vi "PathOff.vi"(11 "Path":T2) -> (3 "PathOut":T2)   [LabVIEW 2014]
uses:
  TypeDefs/Point2DwSlope.ctl
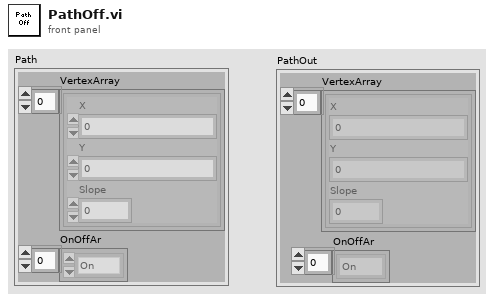
[diagram p1: front panel]
types:
  T1 = typedef "Point2DwSlope.ctl" = cluster{"X":sgl, "Y":sgl, "Slope":dbl}
  T2 = cluster{"VertexArray":T1[], "OnOffAr":enum16{"On", "Off"}[]}
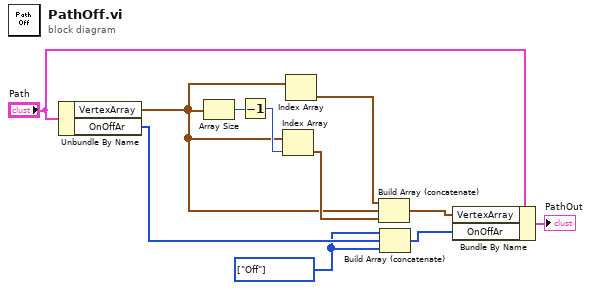
[diagram p0: block diagram]
diagram:
  w1 = enum16{"On", "Off"}[] [enum."Off"] items=["On", "Off"] ("element")
  n1 = Unbundle By Name("Path") -> ("VertexArray"=w3:T1[], "OnOffAr"=w8:enum16{"On", "Off"}[])
  n2 = Array Size(array=w3) -> (size(s)=w11:i32)
  n3 = Decrement(x=w11) -> (x-1=w10:i32)
  n4 = Index Array(array=w3, index=w10) -> (element=w9:T1)
  n5 = Index Array(array=w3) -> (element=w2:T1)  [unwired: 1 in]
  n6 = Build Array (concatenate)(w2, w3, w9) -> (w6:T1[])
  n7 = Build Array (concatenate)(w1, w8, w1) -> (w5:enum16{"On", "Off"}[])
  n8 = Bundle By Name(cluster="Path", "VertexArray"=w6, "OnOffAr"=w5) -> (→"PathOut":T2)
